vi "Display Hologram.vi"() -> (0 "Currant Holo":u8[][](graph))   [LabVIEW 2020]
uses:
  _globals/OpticalPrime Controls.vi
panel:
  in  "Close":bool
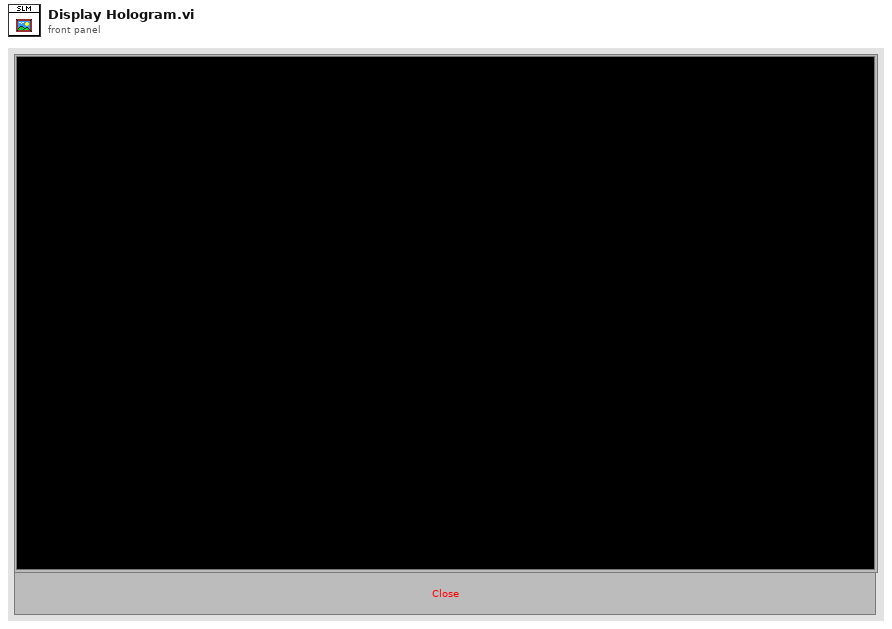
[diagram p1: front panel]
types:
  T1 = typedef "PCIe SLM params.ctl" = cluster{"Width":dbl, "Height":dbl, "Board ID":i32, "Centre Y":dbl, "Centre X":dbl}
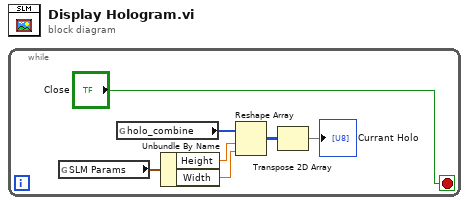
[diagram p0: block diagram]
diagram:
  n1 = while {
    stop <- "Close" stop-if-true
    n2 = global read "OpticalPrime Controls.vi" "SLM Params"() -> (w4:T1)
    n3 = global read "OpticalPrime Controls.vi" "holo_combine"() -> (w5:u8[])
    n4 = Unbundle By Name(w4) -> ("Height"=w6:dbl, "Width"=w7:dbl)
    n5 = Reshape Array(w5, w6, w7) -> (w3:u8[][])
    n6 = Transpose 2D Array(2D array=w3) -> (transposed array=→"Currant Holo":u8[][])
  }
